vi "氨氮测量流程.vi"(10 "量程模式":T1, 11 "参数":T2={"站号"=1, "量程切换"=enum."AUTO", "控制命令"=enum."启动测量", "模式设置"=enum."待机", "测量间隔"=0} {"站号" items=["总磷"=1, "总氮"=2]}) -> ()   [LabVIEW 2016, in "氨氮.lvlib"]
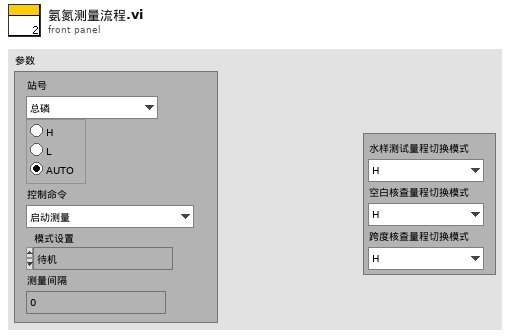
[diagram p1: front panel]
types:
  T1 = cluster{"水样测试量程切换模式":enum16{"H", "L", "AUTO"}, "空白核查量程切换模式":enum16{"H", "L", "AUTO"}, "跨度核查量程切换模式":enum16{"H", "L", "AUTO"}}
  T2 = cluster{"站号":u16, "量程切换":enum32{"H", "L", "AUTO"}, "控制命令":enum16{"启动测量", "标样核查", "零点核查", "跨度核查", "空白测试", "平行样测试", "加标回收", "空白校准", "标样校准", "初始化（清洗）", "停止测试", "仪器重启", "校时", "模式设置", "测量间隔设置"}, "模式设置":enum16{"待机", "连续模式", "周期模式", "定点模式", "受控模式", "手动模式"}, "测量间隔":u16}
  T3 = enum16{"初始化", "通电", "参数1启动", "等待参数1测试完成", "参数1测试完成", "参数1存储数据", "参数2启动", "等待参数2测试完成", "参数2测试完成", "参数2存储数据", "断电", "结束"}
  T4 = cluster{"时间标识":timestamp, "设备":string, "日志信息":string, "流程参数":string}
  T5 = cluster{"时间标识":timestamp, "监测值":sgl, "单位":u16, "数据标识":string, "因子编码":u32, "标样参考值":sgl, "F0":sgl, "F1":sgl, "F2":sgl, "F3":sgl, "温度":sgl, "湿度":sgl, "量程标识":string}
  T6 = enum16{"维护数据", "水样测试", "标样核查", "零点核查", "跨度核查", "空白测试", "平行样测试", "加标回收", "空白校准", "标样校准", "初始化（清洗）"}
  T7 = cluster{"系统时间":timestamp, "工作状态":enum16{"空闲", "水样测试", "标样核查", "零点核查", "跨度核查", "空白测试", "平行样测试", "加标回收", "空白校准", "标样校准", "初始化（清洗）"}, "测量模式":enum16{"待机", "连续模式", "周期模式", "定点模式", "受控模式", "手动模式"}, "告警代码":enum16{"无告警", "缺试剂告警", "缺水样告警", "缺蒸馏水告警", "缺标液告警", "仪表漏液告警", "标定异常告警", "超量程告警", "加热异常", "低试剂预警", "超上限告警", "超下限告警", "仪表内部其他异常", "滴定异常告警", "电极异常告警", "量程切换告警", "参数设置告警", "PH电极电位异常", "电导率电极异常", "浊度光度异常", "溶解氧电极异常", "溶解氧光强异常", "温度异常告警", "PH异常告警", "溶解氧异常告警", "电导率异常告警", "浊度异常告警", "叶绿素异常告警", "藻密度异常告警", "蓝绿藻异常告警", "ORP异常告警", "氨氮异常告警", "清洁刷异常告警", "SD卡异常告警", "蓝牙异常告警", "Wifi异常告警", "流程异常告警"}, "故障代码":enum16{"无故障", "电机故障", "温度故障", "通讯故障", "滴定故障"}, "日志代码":u16, "软件版本":u16, "F0":sgl, "F1":sgl, "F2":sgl, "F3":sgl, "T":sgl, "H":sgl, "id":u16, "flowid":u16, "量程":u16, "总磷控温温度1":sgl, "营养盐控温温度2":sgl, "ADC":sgl}
  T8 = enum16{"启动测量", "标样核查", "零点核查", "跨度核查", "空白测试", "平行样测试", "加标回收", "空白校准", "标样校准", "初始化（清洗）", "停止测试", "仪器重启", "校时", "模式设置", "测量间隔设置"}
  T9 = enum16{"空闲", "水样测试", "标样核查", "零点核查", "跨度核查", "空白测试", "平行样测试", "加标回收", "空白校准", "标样校准", "初始化（清洗）"}
  T10 = cluster{"跨度值":dbl, "零点标准液浓度":dbl, "跨度标准液浓度":dbl, "标准液标准浓度":dbl}
  T11 = cluster{"因子编码":u32, "单位":u16, "标样参考值":sgl, "水样数据时间":timestamp, "水样实测值":sgl, "水样数据标识":string, "标样数据时间":timestamp, "标样实测值":sgl, "标样数据标识":string, "空白数据时间":timestamp, "空白实测值":sgl, "空白数据标识":string, "零点核查数据时间":timestamp, "零点核查实测值":sgl, "零点核查数据标识":string, "跨度核查数据时间":timestamp, "跨度核查实测值":sgl, "跨度核查数据标识":string, "加标回收数据时间":timestamp, "加标回收实测值":sgl, "加标回收数据标识":string, "平行样数据时间":timestamp, "平行样实测值":sgl, "平行样数据标识":string}
  T12 = cluster{"运行模式":enum16{"维护模式", "常规模式", "应急模式", "质控模式"}}
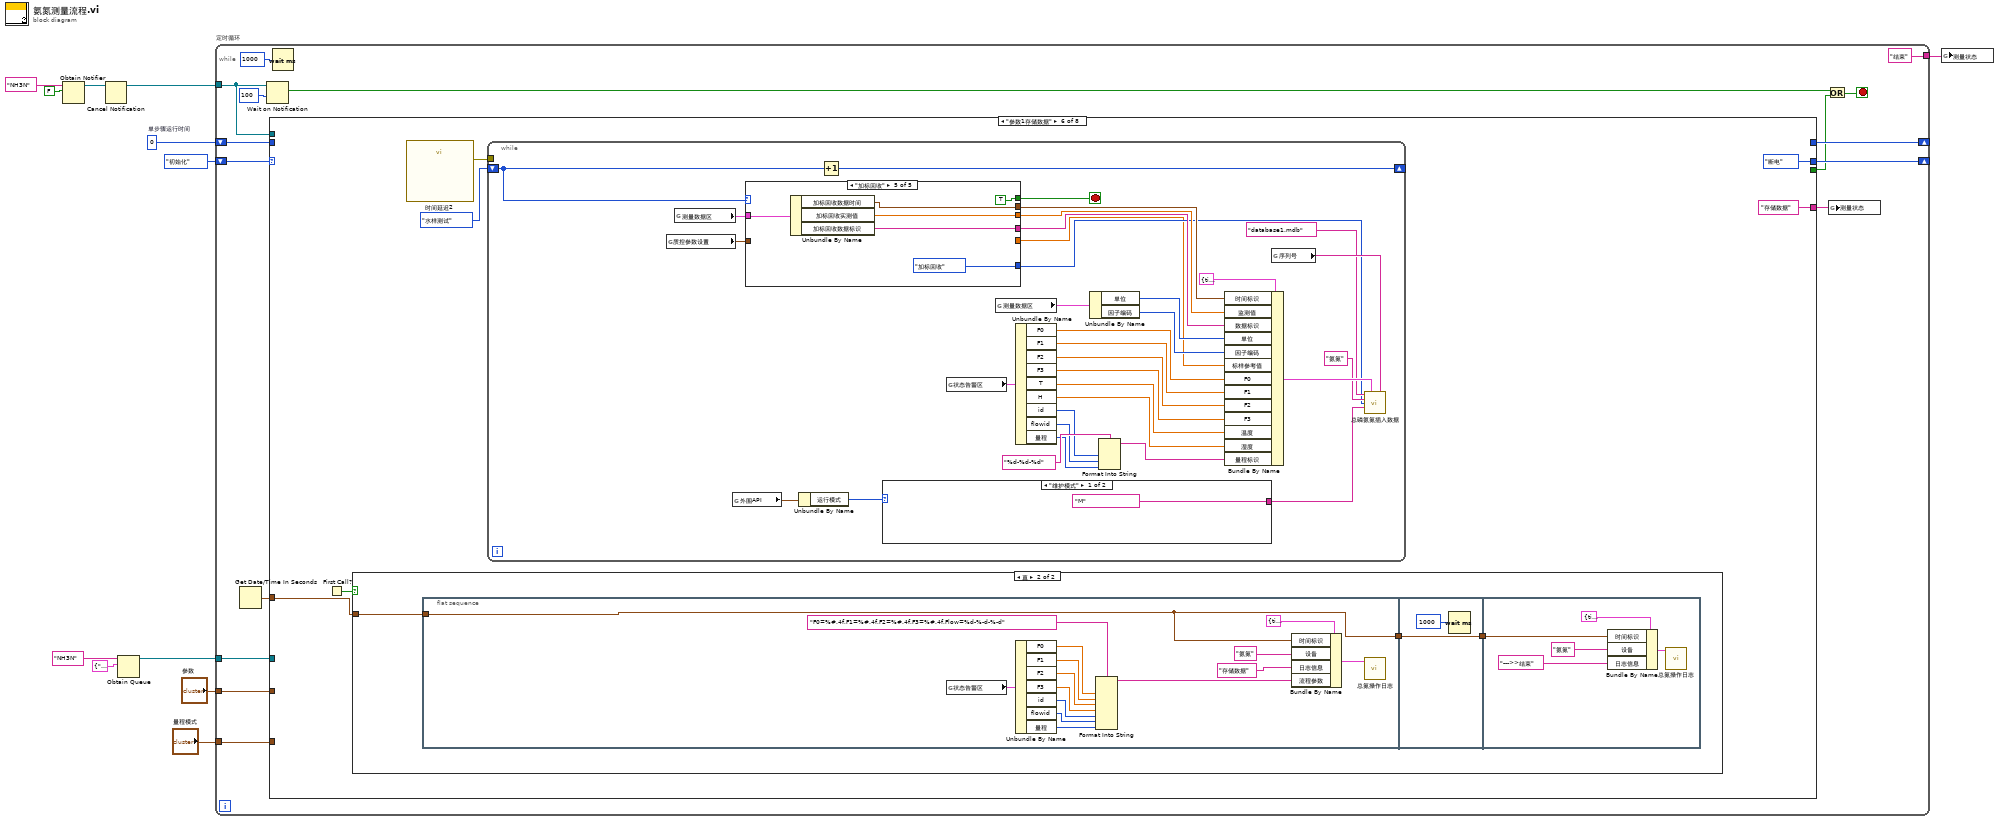
[diagram p0: block diagram]
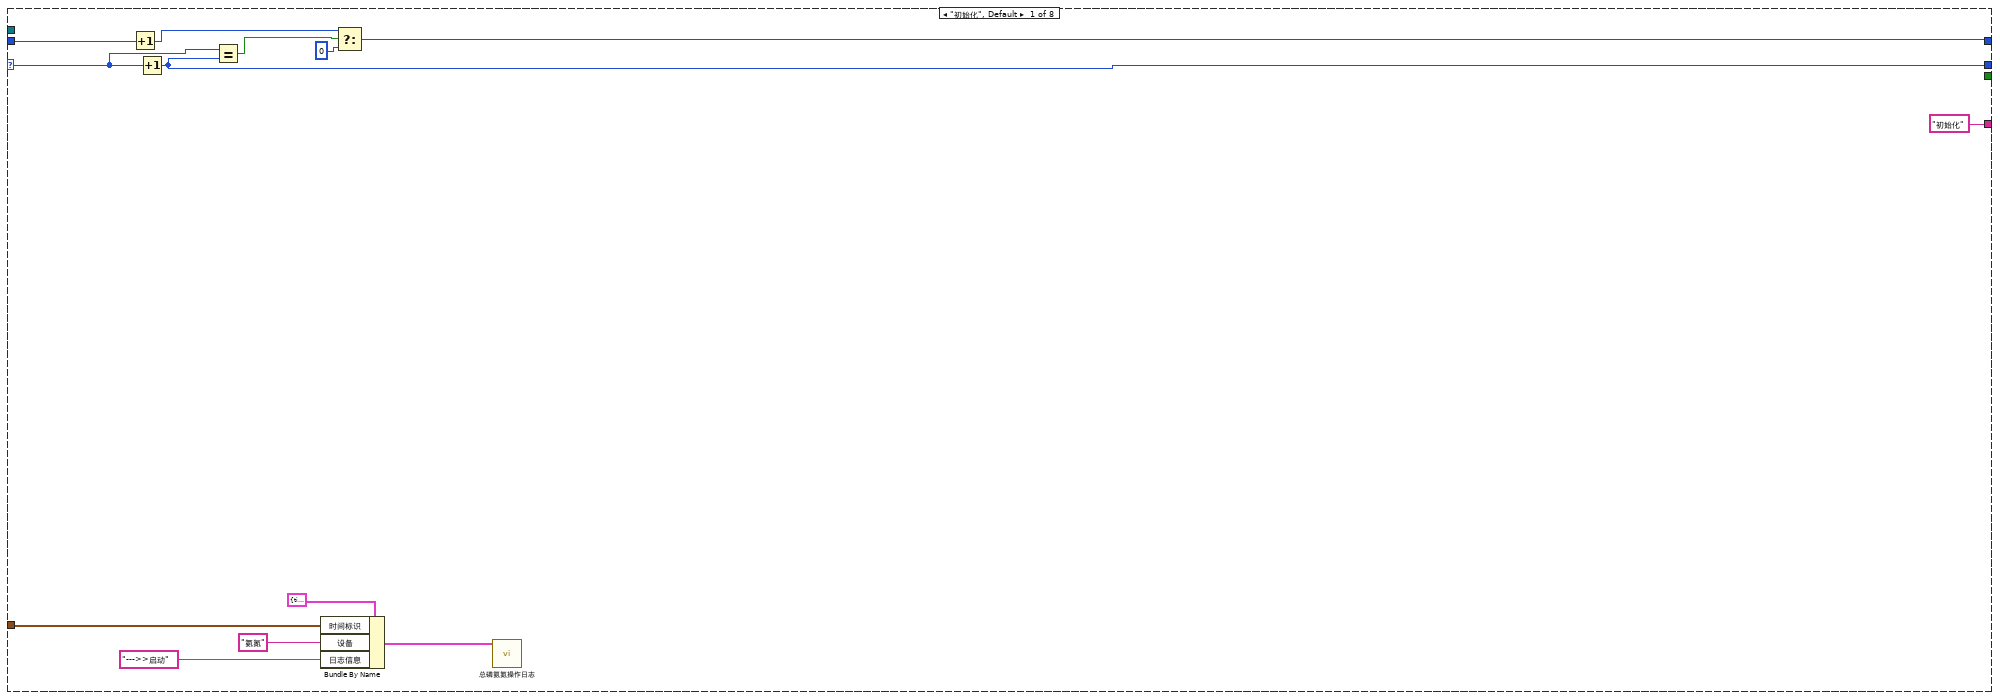
[diagram p2: hidden frame]
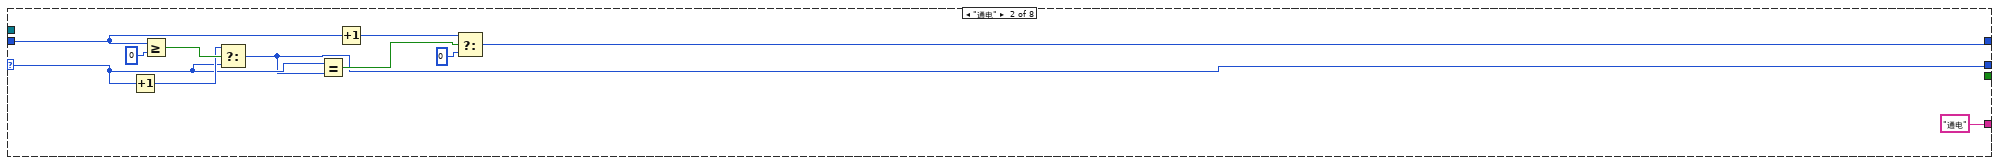
[diagram p3: hidden frame]
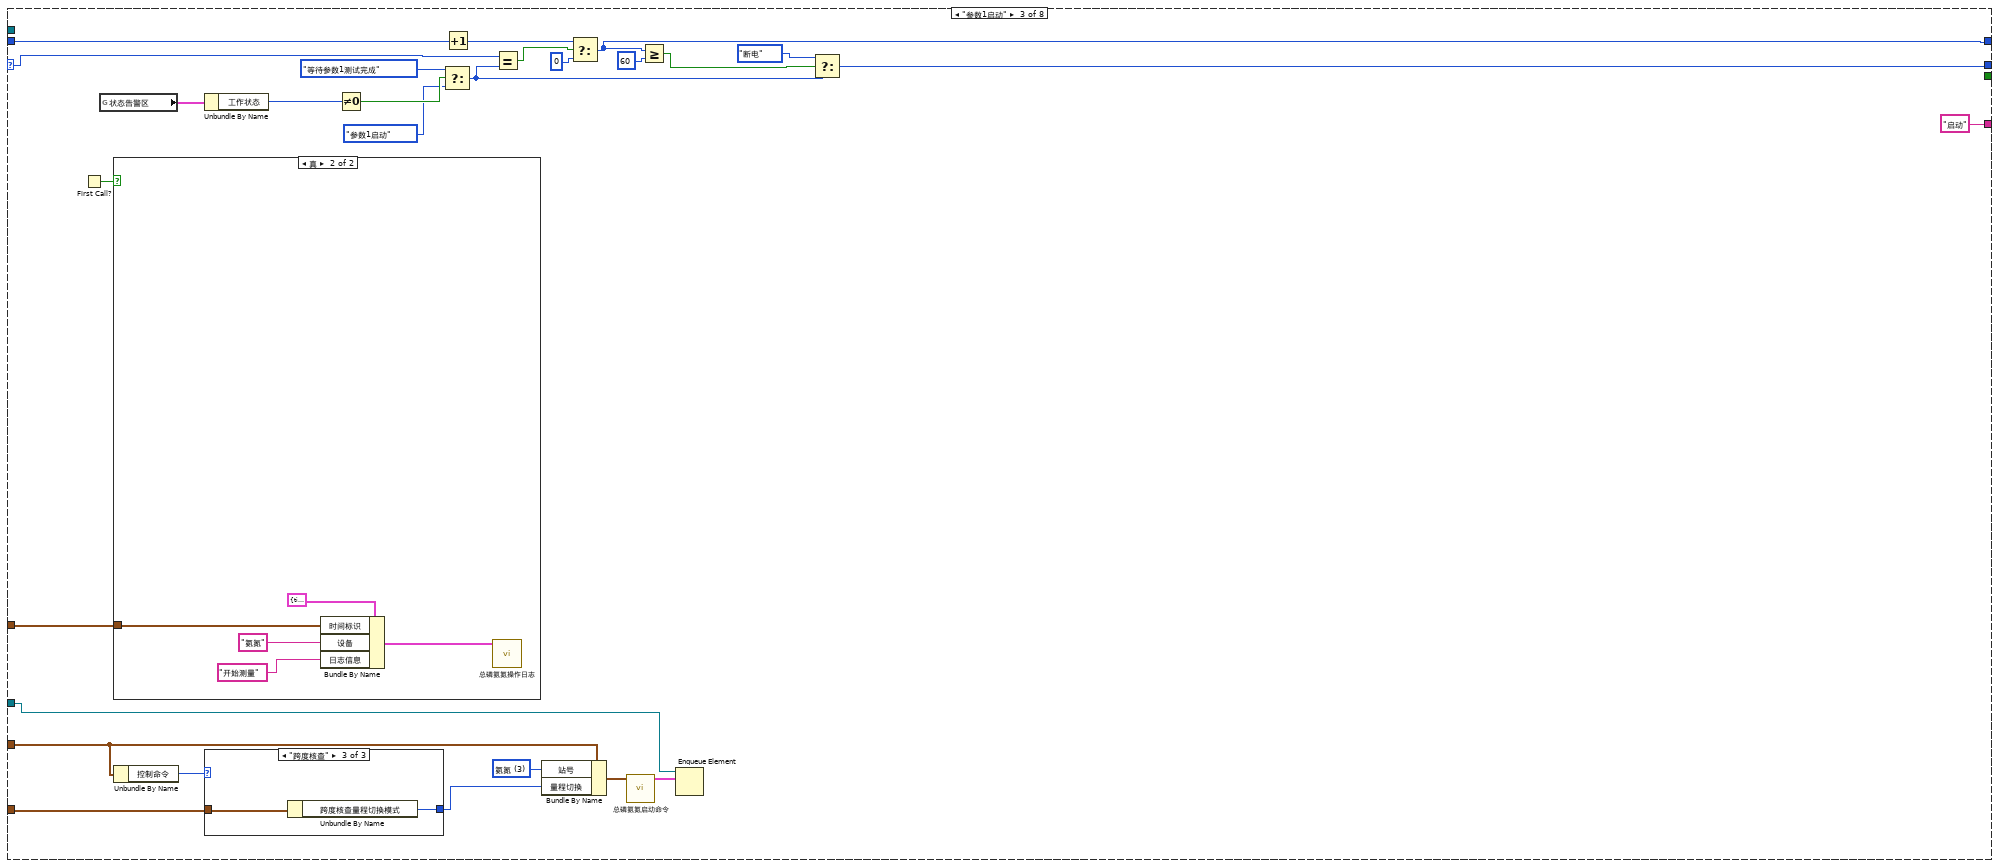
[diagram p4: hidden frame]
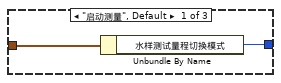
[diagram p5: hidden frame]
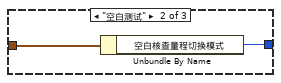
[diagram p6: hidden frame]
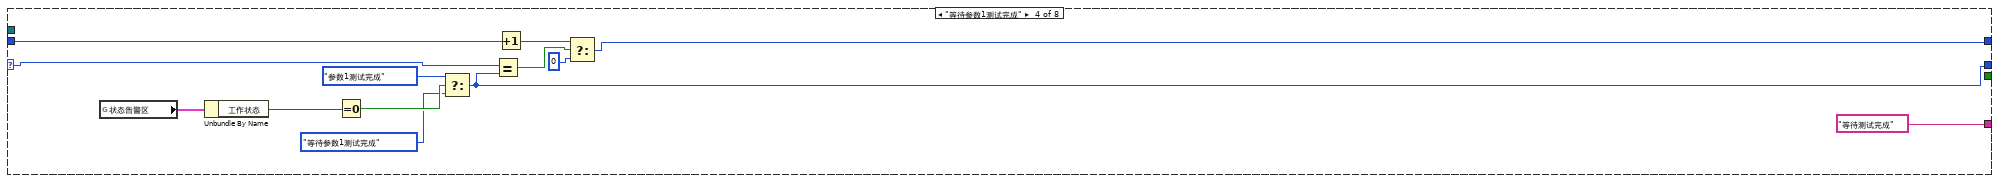
[diagram p8: hidden frame]
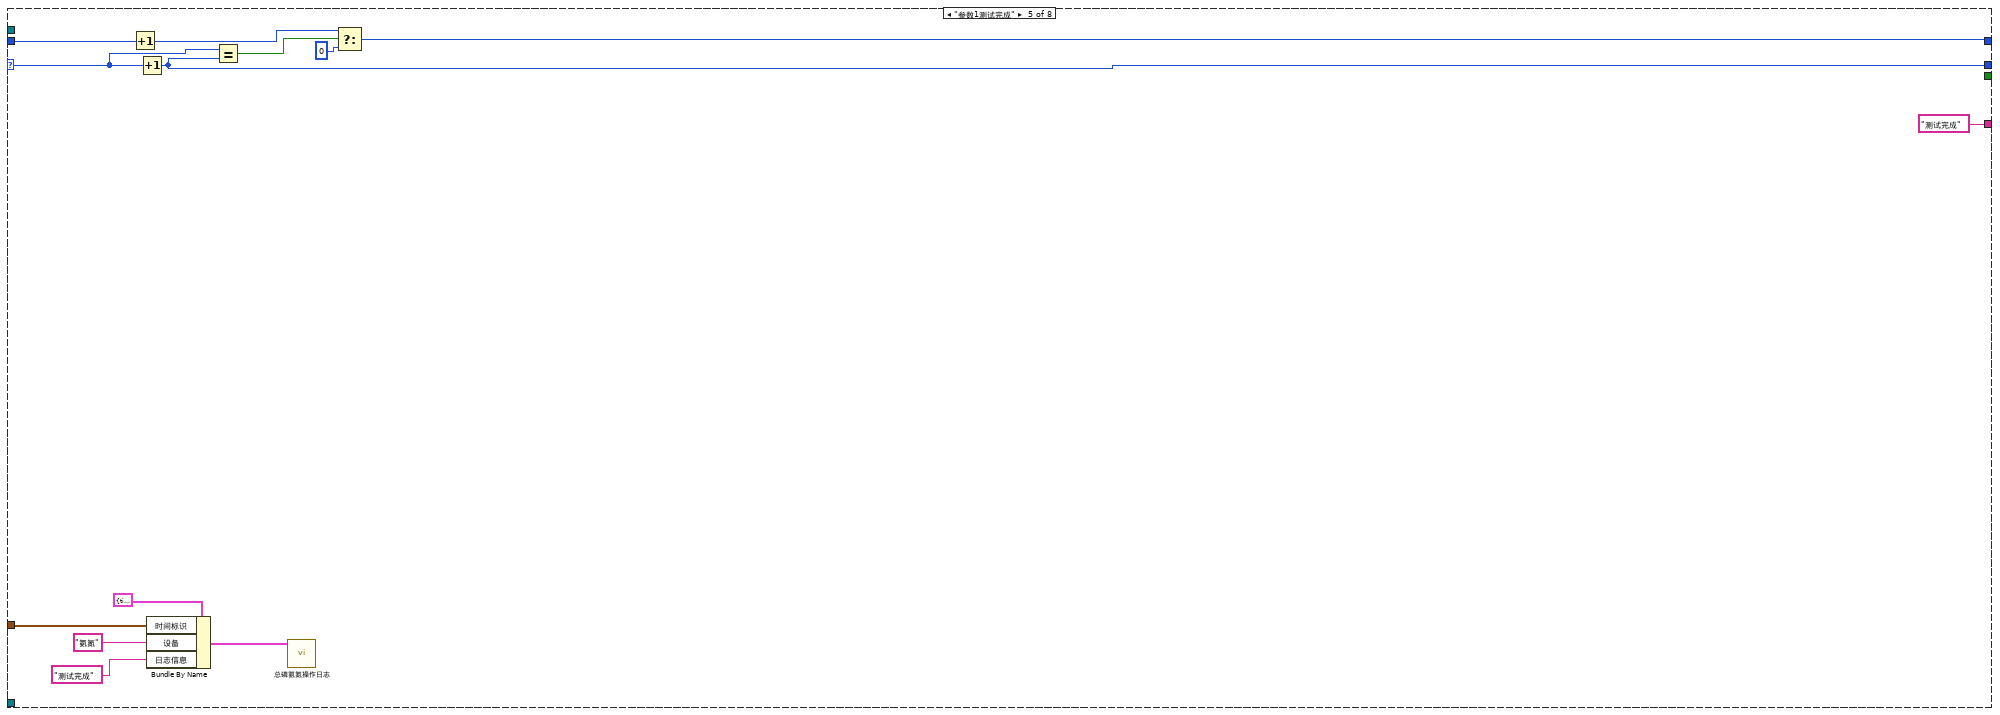
[diagram p9: hidden frame]
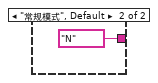
[diagram p10: hidden frame]
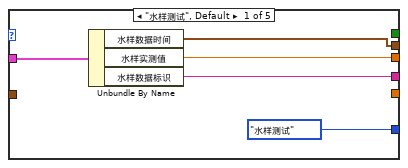
[diagram p11: hidden frame]
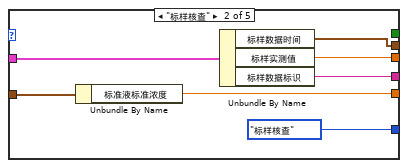
[diagram p12: hidden frame]
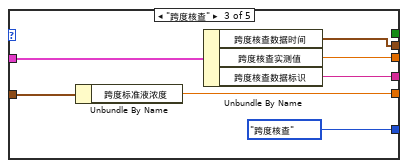
[diagram p13: hidden frame]
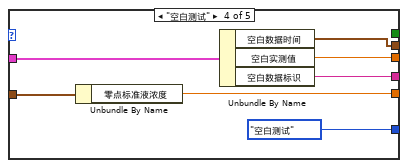
[diagram p14: hidden frame]
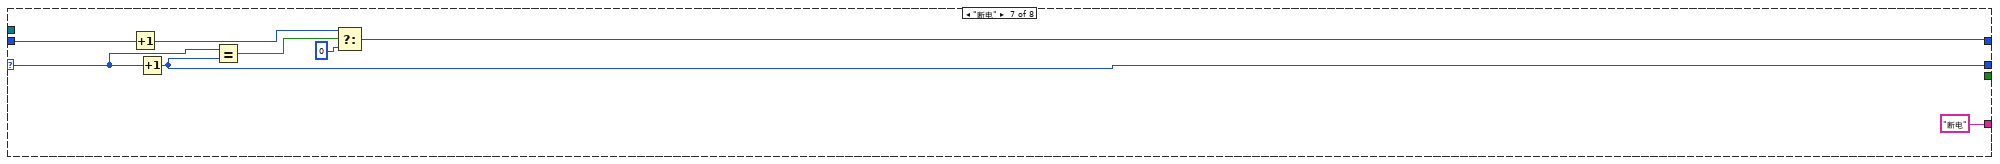
[diagram p16: hidden frame]
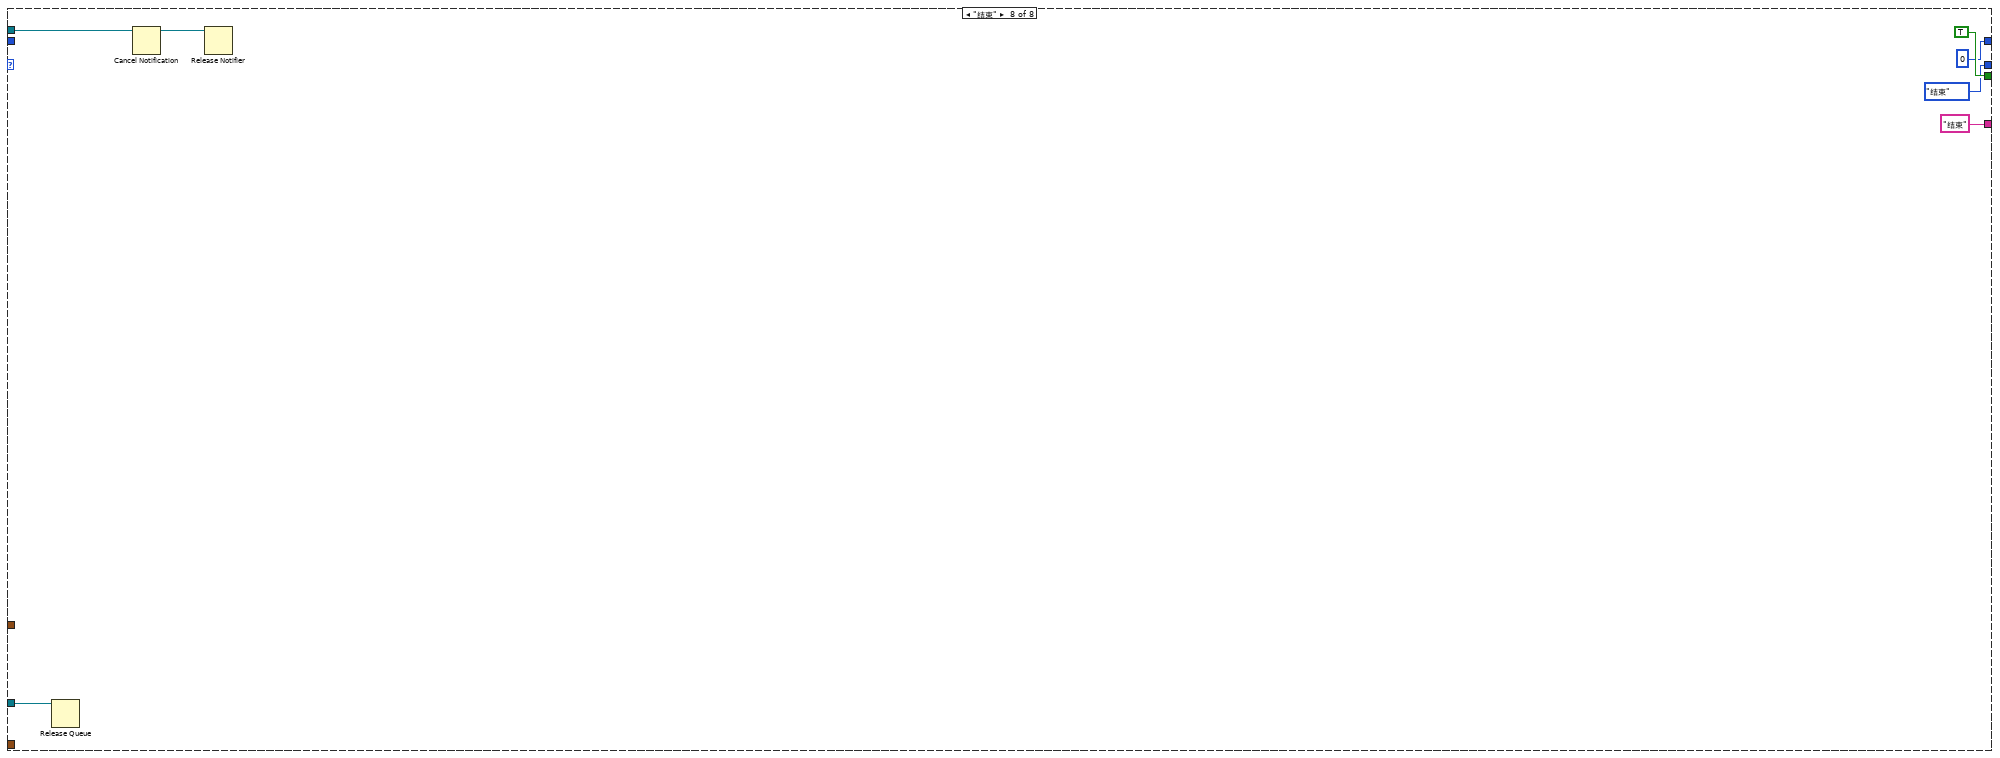
[diagram p17: hidden frame]
diagram:
  w8 = 0  # 单步骤运行时间
  n1 = Obtain Notifier(name (unnamed)="NH3N" ("名称（未命名）"), notification data type=FALSE) -> (notifier out=w5:refnum<notifier>)  [unwired: 2 in, 2 out]
  n2 = Cancel Notification(0:w5) -> (8:w4:refnum<notifier>)  [unwired: 1 in, 2 out]
  n3 = Obtain Queue(name (unnamed)="NH3N" ("名称（未命名）"), element data type=cluster{"命令":string, "data":variant} {"命令"="", "data"=variant}) -> (queue out=w9:refnum<queue>)  [unwired: 3 in, 2 out]
  n4 = while "定时循环" {
    shift-right: [w27] -> _
    shift-left: T3."初始化" ("枚举") -> [w28]
    tunnel: w9 -> [w26]
    shift-right: [w24] -> _
    shift-left: w8 -> [w25]
    tunnel: w4 -> [w23]
    tunnel: "参数" -> [w18]
    tunnel: "量程模式" -> [w15]
    tunnel: ["结束" ("输入 1")] -> w1
    stop <- w19 stop-if-true
    n5 = Get Date/Time In Seconds() -> (seconds since 1Jan1904=w16:timestamp)
    n6 = Wait on Notification(notifier=w23, timeout in ms (-1)=100 ("超时毫秒(-1)")) -> (notification=w20:bool)  [unwired: 2 in, 3 out]
    n7 = case shown="\"参数1存储数据\"" w28 {
      selector: w28 -> [w39 w46 w74 w98 w113 _ w220 _]
      tunnel: [_ _ _ _ _ _ _ TRUE] -> w21
      tunnel: [w40 w45 w56 w97 w112 T3."断电" ("枚举") w219 T3."结束" ("枚举")] -> w27
      tunnel: w26 -> [_ _ w79 _ _ _ _ w227]
      tunnel: w25 -> [w41 w47 w75 w100 w114 _ w222 _]
      tunnel: [w37 w48 w61 w99 w115 _ w221 0 ("t")] -> w24
      tunnel: w23 -> [_ _ _ _ _ _ _ w226]
      tunnel: w18 -> [_ _ w65 _ _ _ _ _]
      tunnel: w16 -> [w31 _ w70 _ w106 w122 _ _]
      tunnel: ["初始化" ("输入 1") "通电" ("输入 1") "启动" ("输入 1") "等待测试完成" ("输入 1") "测试完成" ("输入 1") "存储数据" ("输入 1") "断电" ("输入 1") "结束" ("输入 1")] -> w14
      tunnel: w15 -> [_ _ w63 _ _ _ _ _]
      frame "初始化", Default {
        n8 = Increment(x=w41) -> (x+1=w35:i32)
        n9 = Increment(x=w39) -> (x+1=w40:T3)
        n10 = Equal?(x=w39, y=w40) -> (x = y?=w38:bool)
        n11 = Bundle By Name(cluster=T4 {"时间标识"=timestamp(0 s since 1904-01-01), "设备"="", "日志信息"="", "流程参数"=""} ("data in"), "时间标识"=w31, "设备"="氨氮", "日志信息"="--->>启动") -> (w29:T4)
        n12 = Select(t=w35, s=w38, f=0 ("t")) -> (s? t:f=w37:i32)
        n13 = call "总磷氨氮操作日志.vi"("data in"=w29) -> ()  [unwired: 11 in]
      }
      frame "通电" {
        n14 = Increment(x=w46) -> (x+1=w50:T3)
        n15 = Greater Or Equal?(x=w47, y=0) -> (x >= y?=w51:bool)
        n16 = Select(t=w50, s=w51, f=w46) -> (s? t:f=w45:T3)
        n17 = Equal?(x=w46, y=w45) -> (x = y?=w49:bool)
        n18 = Increment(x=w47) -> (x+1=w44:i32)
        n19 = Select(t=w44, s=w49, f=0 ("t")) -> (s? t:f=w48:i32)
      }
      frame "参数1启动" {
        w71 = u16 3 items=["总磷"=1, "总氮"=2, "氨氮"=3] ("站号")
        n20 = First Call?() -> (First Call?: T/F=w69:bool)
        n21 = global read "VAR总磷氨氮全局变量.vi" "状态告警区"() -> (w53:T7)
        n22 = case shown="真" w69 {
          tunnel: w70 -> [_ w87]
          frame False {
          }
          frame True {
            n23 = Bundle By Name(cluster=T4 {"时间标识"=timestamp(0 s since 1904-01-01), "设备"="", "日志信息"="", "流程参数"=""} ("data in"), "时间标识"=w87, "设备"="氨氮", "日志信息"="开始测量") -> (w86:T4)
            n24 = call "总磷氨氮操作日志.vi"("data in"=w86) -> ()  [unwired: 11 in]
          }
        }
        n25 = Unbundle By Name(w65) -> ("控制命令"=w64:T8)
        n26 = Unbundle By Name(w53) -> ("工作状态"=w78:T9)
        n27 = case shown="\"跨度核查\"" w64 {
          tunnel: w63 -> [w81 w83 w85]
          tunnel: [w80 w82 w84] -> w62
          frame "启动测量", Default {
            n28 = Unbundle By Name(w81) -> ("水样测试量程切换模式"=w80:enum16{"H", "L", "AUTO"})
          }
          frame "空白测试" {
            n29 = Unbundle By Name(w83) -> ("空白核查量程切换模式"=w82:enum16{"H", "L", "AUTO"})
          }
          frame "跨度核查" {
            n30 = Unbundle By Name(w85) -> ("跨度核查量程切换模式"=w84:enum16{"H", "L", "AUTO"})
          }
        }
        n31 = Not Equal To 0?(x=w78) -> (x != 0?=w77:bool)
        n32 = Select(t=T3."等待参数1测试完成" ("枚举"), s=w77, f=T3."参数1启动" ("枚举")) -> (s? t:f=w58:T3)
        n33 = Increment(x=w75) -> (x+1=w72:i32)
        n34 = Equal?(x=w74, y=w58) -> (x = y?=w76:bool)
        n35 = Bundle By Name(cluster=w65, "站号"=w71, "量程切换"=w62) -> (w55:T2)
        n36 = Select(t=w72, s=w76, f=0 ("t")) -> (s? t:f=w61:i32)
        n37 = call "总磷氨氮启动命令.vi"("参数"=w55) -> ("启动命令"=w54:cluster{"命令":string, "data":variant})  [unwired: 10 in]
        n38 = Greater Or Equal?(x=w61, y=60) -> (x >= y?=w59:bool)
        n39 = Enqueue Element(queue=w79, element=w54) -> ()  [unwired: 2 in, 3 out]
        n40 = Select(t=T3."断电" ("枚举"), s=w59, f=w58) -> (s? t:f=w56:T3)
      }
      frame "等待参数1测试完成" {
        n41 = global read "VAR总磷氨氮全局变量.vi" "状态告警区"() -> (w91:T7)
        n42 = Unbundle By Name(w91) -> ("工作状态"=w103:T9)
        n43 = Equal To 0?(x=w103) -> (x = 0?=w102:bool)
        n44 = Select(t=T3."参数1测试完成" ("枚举"), s=w102, f=T3."等待参数1测试完成" ("枚举")) -> (s? t:f=w97:T3)
        n45 = Equal?(x=w98, y=w97) -> (x = y?=w101:bool)
        n46 = Increment(x=w100) -> (x+1=w95:i32)
        n47 = Select(t=w95, s=w101, f=0 ("t")) -> (s? t:f=w99:i32)
      }
      frame "参数1测试完成" {
        n48 = Increment(x=w114) -> (x+1=w110:i32)
        n49 = Increment(x=w113) -> (x+1=w112:T3)
        n50 = Bundle By Name(cluster=T4 {"时间标识"=timestamp(0 s since 1904-01-01), "设备"="", "日志信息"="", "流程参数"=""} ("data in"), "时间标识"=w106, "设备"="氨氮", "日志信息"="测试完成") -> (w104:T4)
        n51 = Equal?(x=w113, y=w112) -> (x = y?=w116:bool)
        n52 = call "总磷氨氮操作日志.vi"("data in"=w104) -> ()  [unwired: 11 in]
        n53 = Select(t=w110, s=w116, f=0 ("t")) -> (s? t:f=w115:i32)
      }
      frame "参数1存储数据" {
        n54 = First Call?() -> (First Call?: T/F=w120:bool)
        n55 = case shown="真" w120 {
          tunnel: w122 -> [_ w192]
          frame False {
          }
          frame True {
            n56 = flat-sequence {
              tunnel: w192 -> [w204]
              tunnel: [w204] -> w191
              tunnel: w191 -> [w209]
              tunnel: [w209] -> w190
              tunnel: w190 -> [w211]
              frame #0 {
                n57 = global read "VAR总磷氨氮全局变量.vi" "状态告警区"() -> (w194:T7)
                n58 = Unbundle By Name(w194) -> ("F0"=w196:sgl, "F1"=w197:sgl, "F2"=w198:sgl, "F3"=w199:sgl, "id"=w200:u16, "flowid"=w201:u16, "量程"=w202:u16)
                n59 = Format Into String(format string="F0=%#.4f,F1=%#.4f,F2=%#.4f,F3=%#.4f,Flow=%d-%-d-%-d" ("格式字符串"), w196, w197, w198, w199, w200, w201, w202) -> (resulting string=w195:string)  [unwired: 2 in, 1 out]
                n60 = Bundle By Name(cluster=T4 {"时间标识"=timestamp(0 s since 1904-01-01), "设备"="", "日志信息"="", "流程参数"=""} ("data in"), "时间标识"=w204, "设备"="氨氮", "日志信息"="存储数据", "流程参数"=w195) -> (w193:T4)
                n61 = call "总氮操作日志.vi"("data in"=w193) -> ()  [unwired: 11 in]
              }
              frame #1 {
                n62 = Wait (ms)(milliseconds to wait=u32 1000 ("等待时间（毫秒）")) -> ()  [unwired: 1 out]
              }
              frame #2 {
                n63 = Bundle By Name(cluster=T4 {"时间标识"=timestamp(0 s since 1904-01-01), "设备"="", "日志信息"="", "流程参数"=""} ("data in"), "时间标识"=w211, "设备"="氨氮", "日志信息"="--->>结束") -> (w210:T4)
                n64 = call "总氮操作日志.vi"("data in"=w210) -> ()  [unwired: 11 in]
              }
            }
          }
        }
        n65 = call "时间延迟2"() -> ("error out"=w117:errorcluster)  [unwired: 11 in]
        n66 = while {
          shift-right: [w149] -> _
          shift-left: enum16{"水样测试", "标样核查", "跨度核查", "空白测试", "加标回收"}."水样测试" ("测量模式") -> [w150]
          tunnel: w117 -> [_]
          stop <- w151 stop-if-true
          n67 = global read "氨氮断电保存全局变量.vi" "质控参数设置"() -> (w124:T10)
          n68 = global read "VAR总磷氨氮全局变量.vi" "测量数据区"() -> (w143:T11)
          n69 = global read "VAR总磷氨氮全局变量.vi" "外围API"() -> (w127:T12)
          n70 = case shown="\"加标回收\"" w150 {
            tunnel: w143 -> [w158 w165 w172 w179 w184]
            tunnel: [w162 w169 w176 w183 w189] -> w148
            tunnel: [w161 w168 w175 w182 w188] -> w147
            tunnel: [w160 w167 w174 w181 w187] -> w146
            tunnel: [T6."水样测试" ("测量模式") T6."标样核查" ("测量模式") T6."跨度核查" ("测量模式") T6."空白测试" ("测量模式") T6."加标回收" ("测量模式")] -> w135
            tunnel: [_ _ _ _ TRUE] -> w151
            tunnel: w124 -> [_ w164 w171 w178 _]
            tunnel: [_ w163 w170 w177 _] -> w123
            frame "水样测试", Default {
              n71 = Unbundle By Name(w158) -> ("水样数据时间"=w162:timestamp, "水样实测值"=w161:sgl, "水样数据标识"=w160:string)
            }
            frame "标样核查" {
              n72 = Unbundle By Name(w164) -> ("标准液标准浓度"=w163:dbl)
              n73 = Unbundle By Name(w165) -> ("标样数据时间"=w169:timestamp, "标样实测值"=w168:sgl, "标样数据标识"=w167:string)
            }
            frame "跨度核查" {
              n74 = Unbundle By Name(w171) -> ("跨度标准液浓度"=w170:dbl)
              n75 = Unbundle By Name(w172) -> ("跨度核查数据时间"=w176:timestamp, "跨度核查实测值"=w175:sgl, "跨度核查数据标识"=w174:string)
            }
            frame "空白测试" {
              n76 = Unbundle By Name(w178) -> ("零点标准液浓度"=w177:dbl)
              n77 = Unbundle By Name(w179) -> ("空白数据时间"=w183:timestamp, "空白实测值"=w182:sgl, "空白数据标识"=w181:string)
            }
            frame "加标回收" {
              n78 = Unbundle By Name(w184) -> ("加标回收数据时间"=w189:timestamp, "加标回收实测值"=w188:sgl, "加标回收数据标识"=w187:string)
            }
          }
          n79 = Unbundle By Name(w127) -> ("运行模式"=w126:enum16{"维护模式", "常规模式", "应急模式", "质控模式"})
          n80 = Increment(x=w150) -> (x+1=w149:enum16{"水样测试", "标样核查", "跨度核查", "空白测试", "加标回收"})
          n81 = case shown="\"维护模式\"" w126 {
            tunnel: ["M" ("数据标记表") "N" ("数据标记表")] -> w125
            frame "维护模式" {
            }
            frame "常规模式", Default {
            }
          }
          n82 = global read "VAR总磷氨氮全局变量.vi" "状态告警区"() -> (w141:T7)
          n83 = global read "VAR总磷氨氮全局变量.vi" "测量数据区"() -> (w142:T11)
          n84 = Unbundle By Name(w141) -> ("F0"=w133:sgl, "F1"=w132:sgl, "F2"=w131:sgl, "F3"=w130:sgl, "T"=w129:sgl, "H"=w128:sgl, "id"=w154:u16, "flowid"=w153:u16, "量程"=w152:u16)
          n85 = Unbundle By Name(w142) -> ("单位"=w145:u16, "因子编码"=w144:u32)
          n86 = Format Into String(format string="%d-%d-%d" ("格式字符串"), w154, w153, w152) -> (resulting string=w134:string)  [unwired: 2 in, 1 out]
          n87 = Bundle By Name(cluster=T5 {"时间标识"=timestamp(0 s since 1904-01-01), "监测值"=0.0, "单位"=0, "数据标识"="", "因子编码"=0, "标样参考值"=0.0, "F0"=0.0, "F1"=0.0, "F2"=0.0, "F3"=0.0, "温度"=0.0, "湿度"=0.0, "量程标识"=""} ("data"), "时间标识"=w148, "监测值"=w147, "数据标识"=w146, "单位"=w145, "因子编码"=w144, "标样参考值"=w123, "F0"=w133, "F1"=w132, "F2"=w131, "F3"=w130, "温度"=w129, "湿度"=w128, "量程标识"=w134) -> (w139:T5)
          n88 = global read "VAR总磷氨氮全局变量.vi" "序列号"() -> (w138:string)
          n89 = call "总磷氨氮插入数据.vi"("database"="database1.mdb", "data"=w139, "SN"=w138, "table"="氨氮", "测量模式"=w135, "数据标记表"=w125) -> ()  [unwired: 9 in, 1 out]
        }
      }
      frame "断电" {
        n90 = Increment(x=w222) -> (x+1=w215:i32)
        n91 = Increment(x=w220) -> (x+1=w219:T3)
        n92 = Equal?(x=w220, y=w219) -> (x = y?=w217:bool)
        n93 = Select(t=w215, s=w217, f=0 ("t")) -> (s? t:f=w221:i32)
      }
      frame "结束" {
        n94 = Release Queue(queue=w227) -> ()  [unwired: 2 in, 3 out]
        n95 = Cancel Notification(0:w226) -> (8:w225:refnum<notifier>)  [unwired: 1 in, 2 out]
        n96 = Release Notifier(notifier=w225) -> ()  [unwired: 2 in, 3 out]
      }
    }
    n97 = Wait (ms)(milliseconds to wait=u32 1000 ("等待时间（毫秒）")) -> ()  [unwired: 1 out]
    n98 = Or(x=w20, y=w21) -> (x .or. y?=w19:bool)
    n99 = global write "VAR总磷氨氮全局变量.vi" "测量状态"(w14) -> ()
  }
  n100 = global write "VAR总磷氨氮全局变量.vi" "测量状态"(w1) -> ()
